vi "SendKeywords.vi"(1 "Strings In":string[](array[string])) -> ()   [LabVIEW 2014]
panel:
  # "This VI gets the telescope keywords and sends them to AzCamServer"
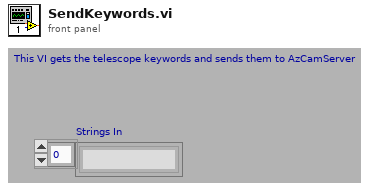
[diagram p1: front panel]
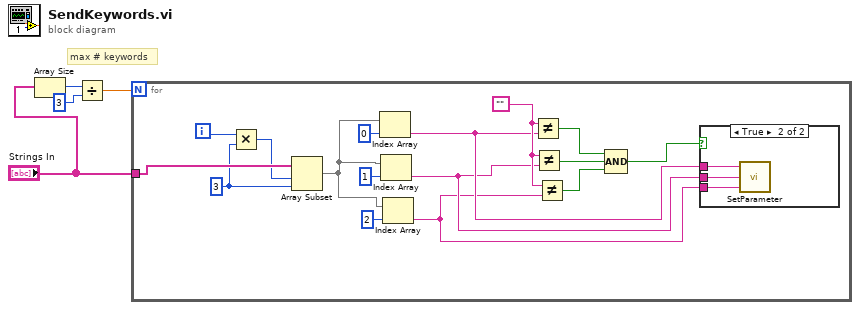
[diagram p0: block diagram]
diagram:
  # "max # keywords"
  n1 = Array Size(array="Strings In") -> (size(s)=w3:i32)
  n2 = Divide(x=w3, y=3) -> (x/y=w1:dbl)
  n3 = for {
    N: w1 -> [_]
    tunnel: "Strings In" -> [w20]
    i -> [w18]
    w11 = ""
    w19 = 3 ("length")
    n4 = Multiply(x=w18, y=w19) -> (x*y=w17:i32)
    n5 = Array Subset(array=w20, index=w17, length=w19) -> (w13:string[])
    n6 = Index Array(array=w13, index=0) -> (element=w7:string)
    n7 = Index Array(array=w13, index=1) -> (element=w6:string)
    n8 = Index Array(array=w13, index=2) -> (element=w5:string)
    n9 = Not Equal?(x=w11, y=w7) -> (x != y?=w12:bool)
    n10 = Not Equal?(x=w11, y=w6) -> (x != y?=w10:bool)
    n11 = Not Equal?(x=w11, y=w5) -> (x != y?=w9:bool)
    n12 = Compound Arithmetic op=AND(w12, w10, w9) -> (w8:bool)
    n13 = case shown="True" w8 {
      tunnel: w7 -> [_ w23]
      tunnel: w6 -> [_ w22]
      tunnel: w5 -> [_ w21]
      frame False {
      }
      frame True {
        n14 = call "SetParameter.vi"("Comment"=w21, "Value"=w22, "Parameter"=w23) -> ()  [unwired: 1 out]
      }
    }
  }
